vi "Configure Internal Trigger.vi"(8 "error in (no error)":errorcluster, 9 "Frequency (100000.0 Hz)":dbl=100000.0, 10 "Channel (1: Channel1)":i32(ring)=1 items=["Channel1"=1, "Channel2"=2], 11 "VISA resource name":refnum<visa-resource-name>) -> (0 "error out":errorcluster, 3 "VISA resource name out":refnum<visa-resource-name>)   [LabVIEW 2012, in "Agilent 81150.lvlib"]
doc: "Configures the internal trigger source.\n\n<B>Note(s):</B>\n(1) This is applicable when the <B>Trigger Source</B> is set to internal."
uses:
  Agilent 81150.lvlib
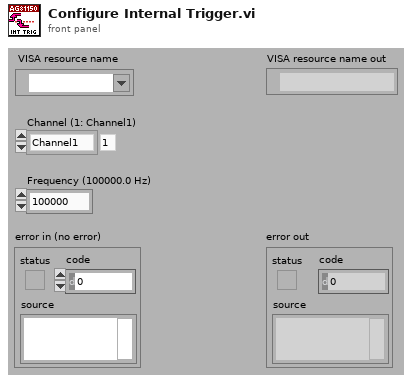
[diagram p1: front panel]
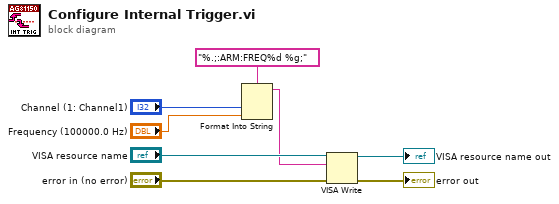
[diagram p0: block diagram]
diagram:
  n1 = Format Into String(format string="%.;:ARM:FREQ%d %g;", "Channel (1: Channel1)", "Frequency (100000.0 Hz)") -> (resulting string=w1:string)  [unwired: 2 in, 1 out]
  n2 = VISA Write(VISA resource name="VISA resource name", write buffer=w1, error in (no error)="error in (no error)") -> (VISA resource name out=→"VISA resource name out":refnum<visa-resource-name>, error out=→"error out":errorcluster)  [unwired: 1 out]
